vi "Configure Tracking Enabled.vi"(8 "error in (no error)":errorcluster, 9 "Tracking Enabled (F: Off)":bool, 11 "VISA resource name":refnum<visa-resource-name>) -> (0 "error out":errorcluster, 3 "VISA resource name out":refnum<visa-resource-name>)   [LabVIEW 2013]
doc: "Sets whether or not the instrument operates in track mode\n\nNotes:\n\n(1) This VI ONLY applies to models E3646A, E3647A, E3648A, & E3649A"
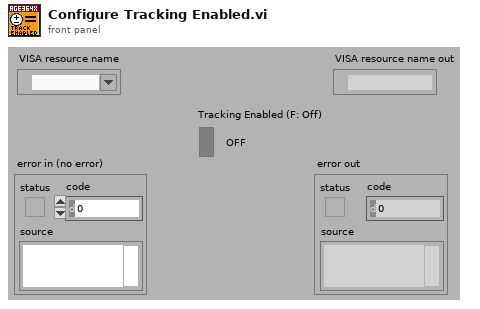
[diagram p1: front panel]
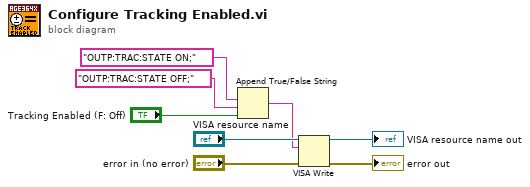
[diagram p0: block diagram]
diagram:
  n1 = Append True/False String(1:"Tracking Enabled (F: Off)", 2:"OUTP:TRAC:STATE OFF;" ("false string"), 3:"OUTP:TRAC:STATE ON;" ("true string")) -> (0:w1:string)  [unwired: 1 in]
  n2 = VISA Write(VISA resource name="VISA resource name", write buffer=w1, error in (no error)="error in (no error)") -> (VISA resource name out=→"VISA resource name out":refnum<visa-resource-name>, error out=→"error out":errorcluster)  [unwired: 1 out]
